vi "TimedDoor_Implement.vi"(11 "ClassThatImplements":refnum<class "TimedDoor.lvclass">) -> (3 "InterfaceHelpClass":refnum<class "TimedDoor_ITimerTimeout.lvclass">)   [LabVIEW 2020, in "TimedDoor_ITimerTimeout.lvclass"]
doc: "Implemnts an Interface"
uses:
  TimedDoor_ITimerTimeout.lvclass
  TimedDoor_class/TimedDoor.lvclass
  TimedDoor_ITimerTimeout.lvclass/TimedDoor_ITimerTimeout.ctl
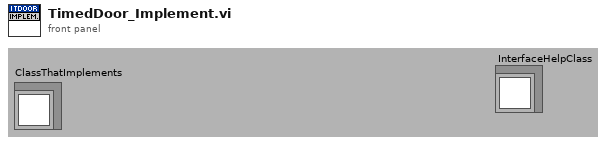
[diagram p1: front panel]
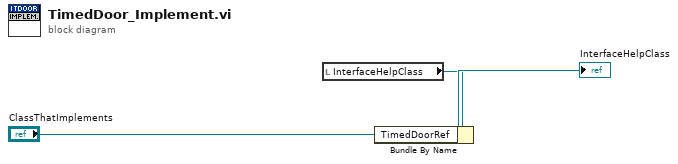
[diagram p0: block diagram]
diagram:
  n1 = local read "InterfaceHelpClass"() -> (w1:refnum<class "TimedDoor_ITimerTimeout.lvclass">)
  n2 = Bundle By Name(cluster=w1, "TimedDoorRef"="ClassThatImplements") -> (→"InterfaceHelpClass":refnum<class "TimedDoor_ITimerTimeout.lvclass">)
